vi "Fix Array Name.vi"(4 "Name":string) -> (7 "Fixed Name":string)   [LabVIEW 2020, in "CDM-Config.lvlib" / "Config Element.lvclass"]
uses:
  Config Element.lvclass
  Config Element.lvclass/Config Element.ctl
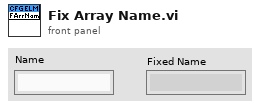
[diagram p1: front panel]
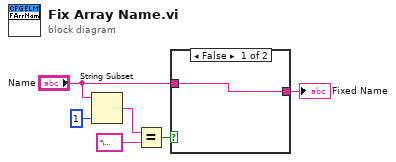
[diagram p0: block diagram]
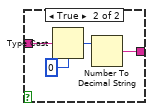
[diagram p2: hidden frame]
diagram:
  n1 = String Subset(string="Name", length (rest)=1 ("length (rest)")) -> (substring=w5:string)  [unwired: 1 in]
  n2 = Equal?(x=w5, y="\u0000") -> (x = y?=w3:bool)
  n3 = case shown="False" w3 {
    tunnel: "Name" -> [w7 w9]
    tunnel: [w7 w8] -> w1
    frame False {
    }
    frame True {
      n4 = Type Cast(type=0, x=w9) -> (*(type *) &x=w11:i32)
      n5 = Number To Decimal String(number=w11) -> (decimal integer string=w8:string)  [unwired: 1 in]
    }
  }
  "Fixed Name" <- w1
